vi "Interpolation Test.vi"() -> ()   [LabVIEW 2018]
uses:
  <vilib>/gmath/NI_Gmath.lvlib
panel:
  out "Array":bool[](array[boolean])
  out "XY Graph":cluster{dbl[], dbl[]}[](graph)
  out "xi used":dbl[](array[numeric]) format="%_6g"
  out "yi":dbl[](array[numeric]) format="%_6g"
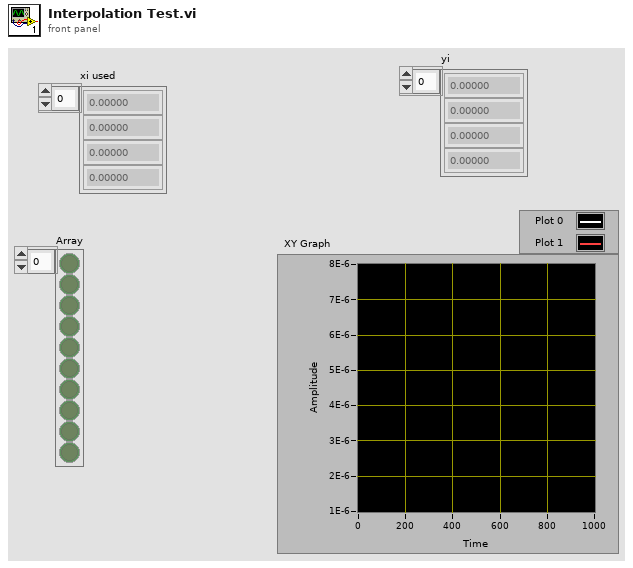
[diagram p1: front panel]
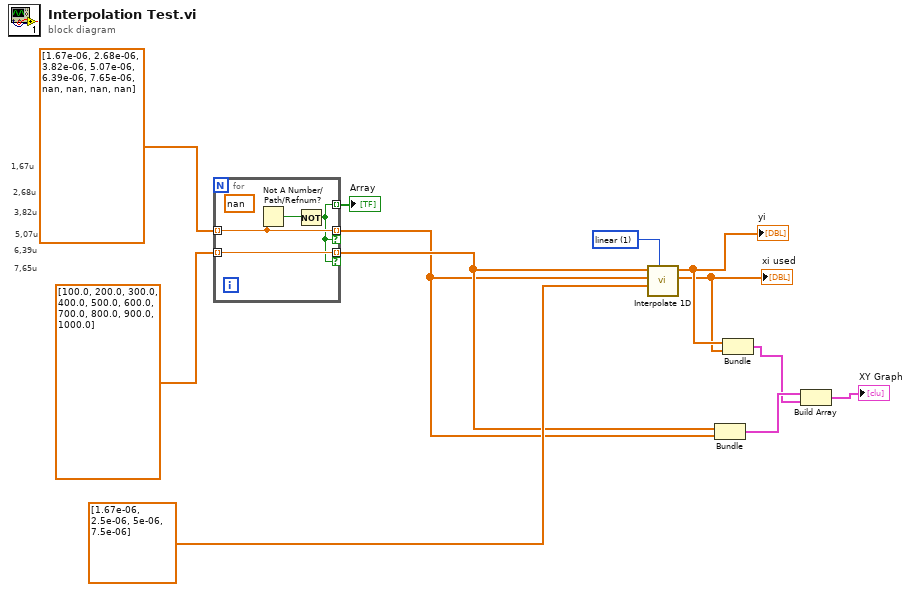
[diagram p0: block diagram]
diagram:
  w11 = 1 items=["nearest", "linear", "spline", "cubic Hermite", "Lagrange"] ("method")
  # "2,68u"
  # "6,39u"
  # "3,82u"
  # "5,07u"
  # "7,65u"
  # "1,67u"
  n1 = for {
    tunnel: dbl[] [1.67e-06, 2.68e-06, 3.82e-06, 5.07e-06, 6.39e-06, 7.65e-06, nan, nan, nan, nan] -> [w15] mode=indexing
    tunnel: dbl[] [100.0, 200.0, 300.0, 400.0, 500.0, 600.0, 700.0, 800.0, 900.0, 1000.0] -> [w16] mode=indexing
    tunnel: [w15] -> w2 mode=indexing if=w13
    tunnel: [w16] -> w3 mode=indexing if=w13
    tunnel: [w13] -> w1 mode=indexing
    (unwired) nan ("x")
    n2 = Not A Number/Path/Refnum?(number/path/refnum=w15) -> (NaN/Path/Refnum?=w14:bool)
    n3 = Not(x=w14) -> (.not. x?=w13:bool)
  }
  "Array" <- w1
  n4 = call <vilib>:"Interpolate 1D.vi"("method"=w11, "xi"=dbl[] [1.67e-06, 2.5e-06, 5e-06, 7.5e-06], "X"=w2, "Y"=w3) -> ("xi used"=w6:dbl[], "yi"=w7:dbl[])  [unwired: 5 in, 1 out]
  "yi" <- w7
  "xi used" <- w6
  n5 = Bundle(w3, w2) -> (w10:cluster{dbl[], dbl[]})  [unwired: 1 in]
  n6 = Bundle("yi"=w7, "xi used"=w6) -> (w8:cluster{"yi":dbl[], "xi used":dbl[]})  [unwired: 1 in]
  n7 = Build Array(w10, w8) -> (→"XY Graph":cluster{"yi":dbl[], "xi used":dbl[]}[])
